vi "enumerateStaticDependencies.vi"(8 "error in (no error)":errorcluster, 11 "SMO.A":refnum<class "SMO.ErrorInjection.lvclass">) -> (0 "error out":errorcluster, 2 "Static Dependencies":refnum<class "SMODependency.lvclass">[](array[class]), 3 "SMO.A out":refnum<class "SMO.ErrorInjection.lvclass">)   [LabVIEW 2013, in "SMO.ErrorInjection.lvclass"]
uses:
  SMO.ErrorInjection.lvclass
  src/Dependency/SMODependency.lvclass
  src/SMO/SMO.lvclass
panel:
  # "For instructions on how to use the JKI State Machine Objects, examples and video tutorials, visit:\nhttp://jki.net/state-machine-objects/\n\nJKI State Machine Objects™\nhttp://jki.net/state-machine-objects/\nCopyright (C) 2005-2015, JKI <info@jki.net>\nALL RIGHTS RESERVED"
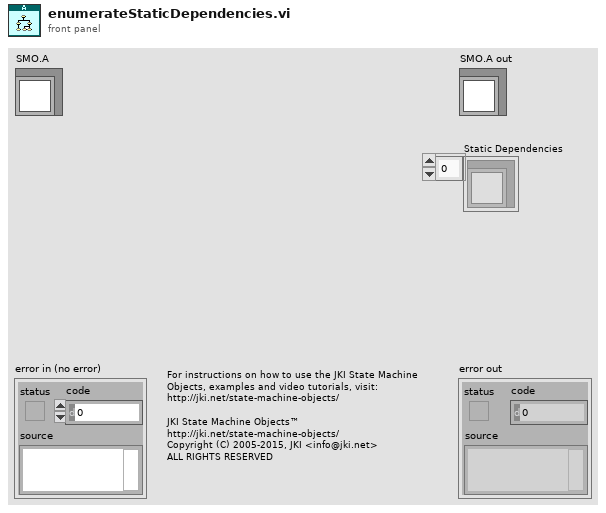
[diagram p1: front panel]
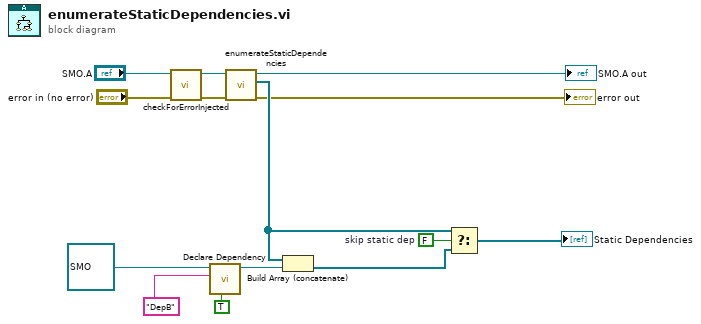
[diagram p0: block diagram]
diagram:
  w11 = FALSE  # skip static dep
  n1 = call "checkForErrorInjected.vi"("error in (no error)"="error in (no error)", "SMO.ErrorInjection in"="SMO.A") -> ("error out"=w5:errorcluster, "SMO.ErrorInjection dup"=w3:refnum<class "SMO.ErrorInjection.lvclass">)  [unwired: 8 in]
  n2 = call "Declare Dependency.vi"("Shared Resource (F)"=TRUE, "Name"="DepB", "Type"=refnum<class "SMO.lvclass"> refnum ("SMO.lvclass")) -> ("Dependency out"=w12:refnum<class "SMODependency.lvclass">)  [unwired: 7 in, 1 out]
  n3 = call-parent "enumerateStaticDependencies.vi"("error in (no error)"=w5, "SMO"=w3) -> ("error out"=→"error out":errorcluster, "Static Dependencies"=w8:refnum<class "SMODependency.lvclass">[], "SMO out"=→"SMO.A out":refnum<class "SMO.ErrorInjection.lvclass">)  [unwired: 7 in]
  n4 = Build Array (concatenate)(w8, w12) -> (w10:refnum<class "SMODependency.lvclass">[])
  n5 = Select(t=w8, s=w11, f=w10) -> (s? t:f=→"Static Dependencies":refnum<class "SMODependency.lvclass">[])
